vi "Tab Demo.vi"() -> ()   [LabVIEW 2018, in "Tab.lvlib"]
uses:
  Tab.lvlib
  Tab Action.ctl
  Tab Refnums.ctl
  Tab Mouse.ctl
  <vilib>/Utility/miscctls.llb/LVPoint32TypeDef.ctl
  Tab Test.vi
  Exit/Exit.lvlib
panel:
  in  "Select":bool
  out "Picture":picture
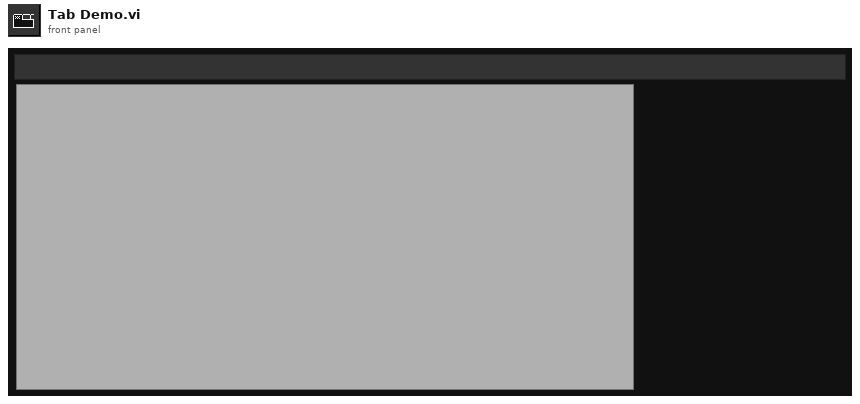
[diagram p1: front panel]
types:
  T1 = typedef "Tab.lvlib/Tab Action.ctl" = enum8{"noop", "new", "init", "close", "start", "render", "tab_add", "tab_change", "tab_hover", "tab_event", "tab_insert", "tab_popout", "tab_close", "theme_change", "resize"}
  T2 = typedef "Tab.lvlib/Tab Refnums.ctl" = cluster{"VI":refnum<vi>, "Picture":refnum<vi>, "Sub Panel":refnum<vi>}
  T3 = typedef "Tab.lvlib/Tab Mouse.ctl" = cluster{"Horizontal":i32, "Vertical":i32, "Button":u16, "Shift":bool, "Ctrl":bool, "Alt":bool, "Double Click":bool}
  T4 = typedef "LVPoint32TypeDef.ctl" = cluster{"Horizontal":i32, "Vertical":i32}
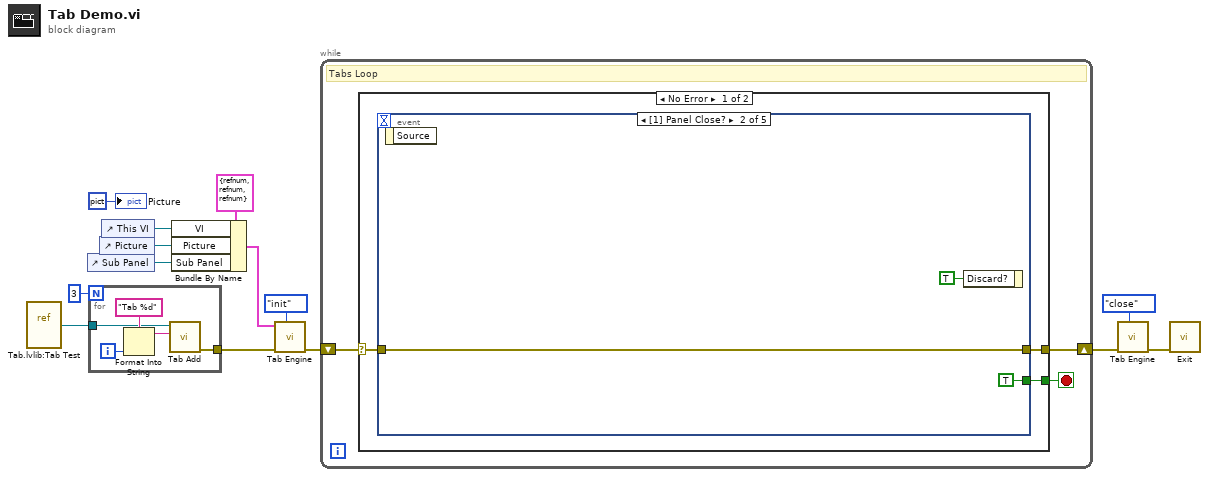
[diagram p0: block diagram]
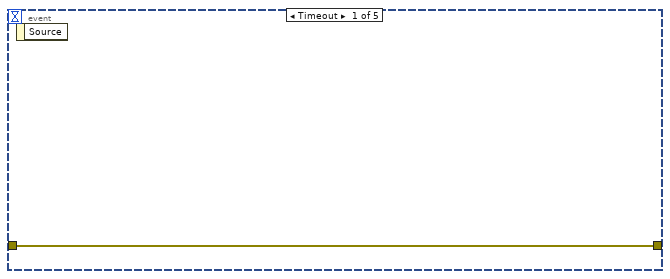
[diagram p2: hidden frame]
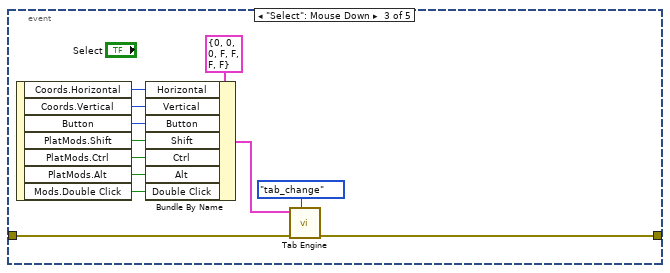
[diagram p3: hidden frame]
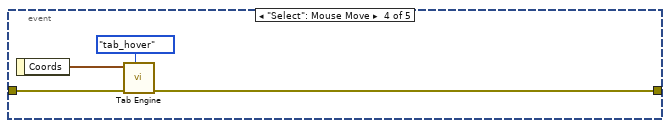
[diagram p4: hidden frame]
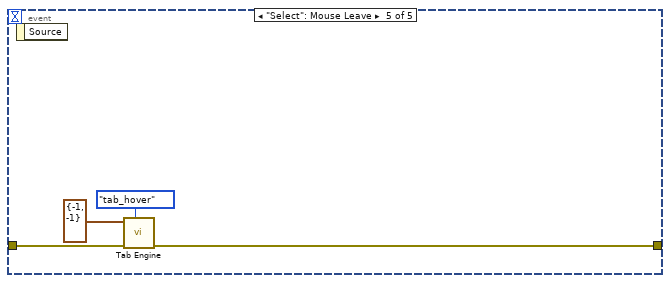
[diagram p5: hidden frame]
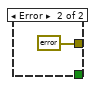
[diagram p6: hidden frame]
diagram:
  n1 = vi-ref "Tab.lvlib:Tab Test.vi"() -> (w4:refnum<vi>)
  n2 = control-ref of="Sub Panel"() -> (w7:refnum<vi>)
  n3 = for {
    N: 3 -> [_]
    tunnel: [w19] -> w6
    tunnel: w4 -> [w15]
    i -> [w18]
    n4 = Format Into String(format string="Tab %d", w18) -> (resulting string=w16:string)  [unwired: 2 in, 1 out]
    n5 = call "Tab Add.vi"("Tab Name"=w16, "VI Refnum"=w15) -> ("error out"=w19:errorcluster)  [unwired: 9 in]
  }
  n6 = control-ref of="Picture"() -> (w11:refnum<vi>)
  n7 = control-ref of="This VI"() -> (w12:refnum<vi>)
  n8 = Bundle By Name(cluster=T2 {"VI"=refnum, "Picture"=refnum, "Sub Panel"=refnum} ("Refnums"), "VI"=w12, "Picture"=w11, "Sub Panel"=w7) -> (w10:T2)
  n9 = call "Tab Engine.vi"("Action"=Tab_Action."init", "error in (no error)"=w6, "Variant in"=w10) -> ("error out"=w2:errorcluster)  [unwired: 7 in, 1 out]
  n10 = while {
    shift-right: [w21] -> w1
    shift-left: w2 -> [w22]
    stop <- w20 stop-if-true
    # "Tabs Loop"
    n11 = case shown="No Error" w22 {
      selector: w22 -> [w25 _]
      tunnel: [w24 errorcluster {"status"=FALSE, "code"=0, "source"=""} ("error IO")] -> w21
      tunnel: [w23 _] -> w20
      frame No Error {
        n12 = event shown="[1] Panel Close?" {
          selector: _ -> [_ _ _ _ _]
          dyn-events: _ -> [_ _ _ _ _]
          timeout: _ -> [_ _ _ _ _]
          tunnel: w25 -> [w26 w27 w32 w44 w48]
          tunnel: [w26 w27 w31 w43 w47] -> w24
          tunnel: [_ TRUE _ _ _] -> w23
          event Timeout {
            n13 = event-data() -> ()  [unwired: 1 in, 1 out]
          }
          event Panel Close? {
            n14 = event-data() -> ()  [unwired: 1 in, 1 out]
            n15 = event-data("Discard?"=TRUE) -> ()  [unwired: 1 in, 1 out]
          }
          event "Select": Mouse Down {
            n16 = event-data() -> ("Coords.Horizontal"=w40:i32, "Coords.Vertical"=w39:i32, "Button"=w38:u16, "PlatMods.Shift"=w37:bool, "PlatMods.Ctrl"=w36:bool, "PlatMods.Alt"=w35:bool, "Mods.Double Click"=w34:bool)  [unwired: 1 in]
            n17 = Bundle By Name(cluster=T3 {"Horizontal"=0, "Vertical"=0, "Button"=0, "Shift"=FALSE, "Ctrl"=FALSE, "Alt"=FALSE, "Double Click"=FALSE} ("Mouse"), "Horizontal"=w40, "Vertical"=w39, "Button"=w38, "Shift"=w37, "Ctrl"=w36, "Alt"=w35, "Double Click"=w34) -> (w30:T3)
            n18 = call "Tab Engine.vi"("Action"=Tab_Action."tab_change", "error in (no error)"=w32, "Variant in"=w30) -> ("error out"=w31:errorcluster)  [unwired: 7 in, 1 out]
          }
          event "Select": Mouse Move {
            n19 = event-data() -> ("Coords"=w42:T4)  [unwired: 1 in]
            n20 = call "Tab Engine.vi"("Action"=Tab_Action."tab_hover", "error in (no error)"=w44, "Variant in"=w42) -> ("error out"=w43:errorcluster)  [unwired: 7 in, 1 out]
          }
          event "Select": Mouse Leave {
            n21 = event-data() -> ()  [unwired: 1 in, 1 out]
            n22 = call "Tab Engine.vi"("Action"=Tab_Action."tab_hover", "error in (no error)"=w48, "Variant in"=T4 {"Horizontal"=-1, "Vertical"=-1} ("Coords")) -> ("error out"=w47:errorcluster)  [unwired: 7 in, 1 out]
          }
        }
      }
      frame Error {
      }
    }
  }
  n23 = call "Tab Engine.vi"("Action"=Tab_Action."close", "error in (no error)"=w1) -> ("error out"=w3:errorcluster)  [unwired: 8 in, 1 out]
  n24 = call "Exit.vi"("error in (no error)"=w3) -> ()  [unwired: 10 in, 1 out]
  "Picture" <- picture data[5B] ("Picture")
